vi "Back.vi"(8 "error in":errorcluster, 11 "Tree":refnum<vi>) -> (0 "error out":errorcluster)   [LabVIEW 2020]
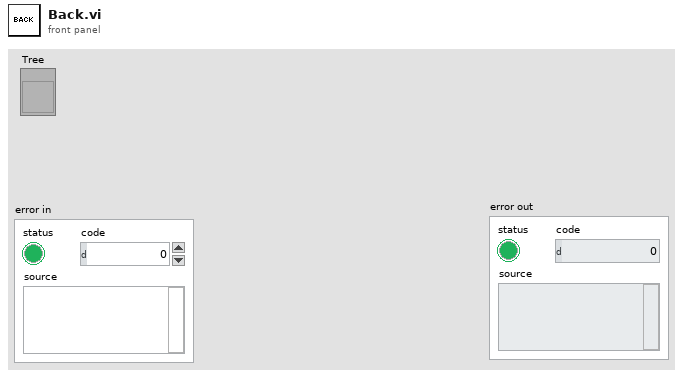
[diagram p1: front panel]
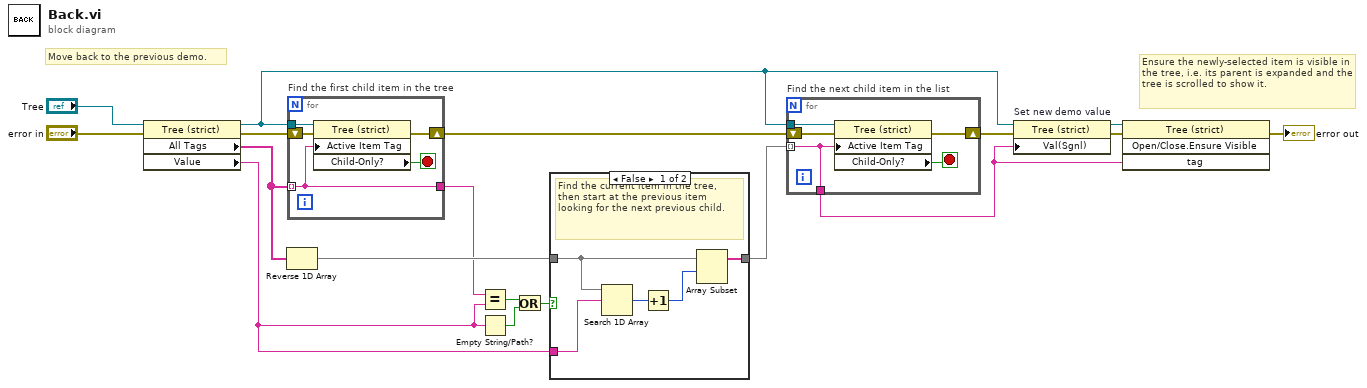
[diagram p0: block diagram]
diagram:
  # "Ensure the newly-selected item is visible in the tree, i.e. its parent is expanded and the tree is scrolled to show it."
  # "Move back to the previous demo."
  n1 = property class="Tree (strict)"(reference="Tree", error in="error in") -> (reference out=w7:refnum<vi>, error out=w9:errorcluster, "All Tags"=w6:string[], "Value"=w12:string)
  n2 = Reverse 1D Array(array=w6) -> (reversed array=w10:string[])
  n3 = for "Find the first child item in the tree" {
    shift-right: [w22] -> w8
    shift-left: w9 -> [w23]
    tunnel: w7 -> [w21]
    tunnel: w6 -> [w20] mode=indexing
    tunnel: [w20] -> w5
    stop <- w19 stop-if-true
    n4 = property class="Tree (strict)"(reference=w21, error in=w23, "Active Item Tag"=w20) -> (error out=w22:errorcluster, "Child-Only?"=w19:bool)  [unwired: 1 out]
  }
  n5 = Equal?(x=w5, y=w12) -> (x = y?=w15:bool)
  n6 = Empty String/Path?(string/path=w12) -> (empty?=w14:bool)
  n7 = Or(x=w15, y=w14) -> (x .or. y?=w13:bool)
  n8 = case shown="False" w13 {
    tunnel: w10 -> [w27 w29]
    tunnel: w12 -> [w28 _]
    tunnel: [w24 w29] -> w11
    frame False {
      # "Find the current item in the tree, then start at the previous item looking for the next previous child."
      n9 = Search 1D Array(1D array=w27, element=w28) -> (index of element=w26:i32)  [unwired: 1 in]
      n10 = Increment(x=w26) -> (x+1=w25:i32)
      n11 = Array Subset(array=w27, index=w25) -> (w24:string[])  [unwired: 1 in]
    }
    frame True {
      # "If there is no item selected in the tree (or the first item is selected), then find the last child item in the tree."
    }
  }
  n12 = for "Find the next child item in the list" {
    shift-right: [w33] -> w17
    shift-left: w8 -> [w34]
    tunnel: w7 -> [w32]
    tunnel: w11 -> [w30] mode=indexing
    tunnel: [w30] -> w1
    stop <- w31 stop-if-true
    n13 = property class="Tree (strict)"(reference=w32, error in=w34, "Active Item Tag"=w30) -> (error out=w33:errorcluster, "Child-Only?"=w31:bool)  [unwired: 1 out]
  }
  n14 = property on="Set new demo value" class="Tree (strict)"(reference=w7, error in=w17, "Val(Sgnl)"=w1) -> (reference out=w3:refnum<vi>, error out=w4:errorcluster)
  n15 = invoke class="Tree (strict)" method="Open/Close.Ensure Visible"(reference=w3, error in=w4, "tag"=w1) -> (error out=→"error out":errorcluster)  [unwired: 1 in, 3 out]
